vi "dfd_Lattice Coef Cluster Validation.vi"(8 "error in (no error)":errorcluster, 11 "Lattice coef":T2) -> (0 "error out":errorcluster, 1 "gain":dbl, 2 "v":dbl[](array[numeric]), 3 "k":dbl[](array[numeric]), 5 "lattice type":T1)   [LabVIEW 2017, in "NI_DigFilterLicensed.lvlib"]
uses:
  <vilib>/addons/Digital Filter Design/NI_DigFilterLicensed.lvlib
  <vilib>/addons/Digital Filter Design/_Objects.llb/DFD Filter Structure Type Selector.ctl
  <vilib>/addons/Digital Filter Design/_Misc.llb/dfd_Error Handlers (Multiple).vi
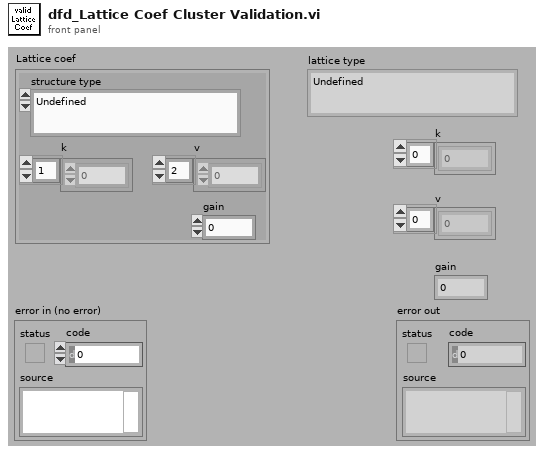
[diagram p1: front panel]
types:
  T1 = typedef "NI_DigFilterLicensed.lvlib/DFD Filter Structure Type Selector.ctl" = enum16{"Undefined", "FIR Direct Form", "FIR Direct Form Transposed", "FIR Symmetric", "FIR Antisymmetric", "IIR Direct Form I", "IIR Direct Form I Transposed", "IIR Direct Form II", "IIR Direct Form II Transposed", "IIR Cascaded Second Order Sections Form I", "IIR Cascaded Second Order Sections Form I Transposed", "IIR Cascaded Second Order Sections Form II", "IIR Cascaded Second Order Sections Form II Transposed", "Lattice Allpass (basic sections)", "Lattice Allpass (one multiplier sections)", "Lattice Allpass (normalized sections)", "Lattice AR (basic sections)", "Lattice AR (one multiplier sections)", "Lattice AR (normalized sections)", "Lattice MA (minimum phase)", "Lattice MA (maximum phase)", "Lattice ARMA (basic sections)", "Lattice ARMA (one multiplier sections)", "Lattice ARMA (normalized sections)"}
  T2 = cluster{"structure type":T1, "k":dbl[], "v":dbl[], "gain":dbl}
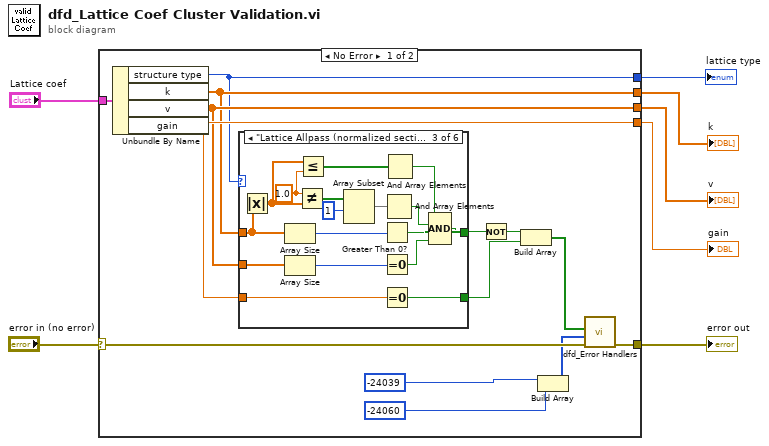
[diagram p0: block diagram]
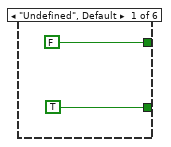
[diagram p2: hidden frame]
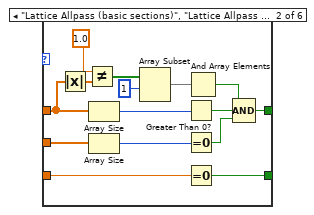
[diagram p3: hidden frame]
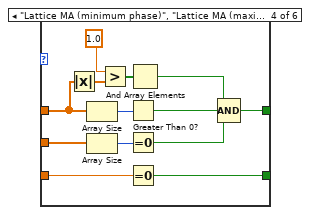
[diagram p4: hidden frame]
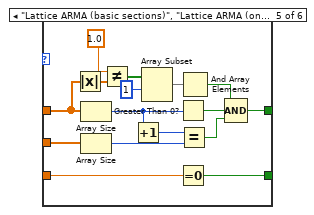
[diagram p5: hidden frame]
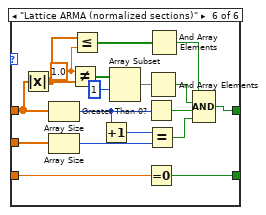
[diagram p6: hidden frame]
diagram:
  n1 = case shown="No Error" "error in (no error)" {
    selector: "error in (no error)" -> [w20 w103]
    tunnel: "Lattice coef" -> [w21 _]
    tunnel: [w19 w103] -> w5
    tunnel: [w18 _] -> w1
    tunnel: [w17 _] -> w2
    tunnel: [w16 _] -> w3
    tunnel: [w15 _] -> w4
    frame No Error {
      n2 = Unbundle By Name(w21) -> ("structure type"=w15:T1, "k"=w16:dbl[], "v"=w17:dbl[], "gain"=w18:dbl)
      n3 = case shown="\"Lattice Allpass (normalized sections)\", \"Lattice AR (normalized sections)\"" w15 {
        tunnel: w16 -> [_ w35 w52 w65 w82 w100]
        tunnel: w17 -> [_ w38 w55 w68 w84 w102]
        tunnel: w18 -> [_ w36 w53 w66 w83 w101]
        tunnel: [FALSE w28 w47 w57 w73 w93] -> w14
        tunnel: [TRUE w24 w43 w56 w69 w89] -> w11
        frame "Undefined", Default {
        }
        frame "Lattice Allpass (basic sections)", "Lattice Allpass (one multiplier sections)", "Lattice AR (basic sections)", "Lattice AR (one multiplier sections)" {
          n4 = Absolute Value(x=w35) -> (abs(x)=w33:dbl[])
          n5 = Not Equal?(x=1.0, y=w33) -> (x != y?=w27:bool[])
          n6 = Array Size(array=w35) -> (size(s)=w34:i32)
          n7 = Array Size(array=w38) -> (size(s)=w37:i32)
          n8 = Array Subset(array=w27, index=1) -> (w25:bool[])  [unwired: 1 in]
          n9 = Greater Than 0?(x=w34) -> (x > 0?=w30:bool)
          n10 = Equal To 0?(x=w37) -> (x = 0?=w31:bool)
          n11 = Equal To 0?(x=w36) -> (x = 0?=w24:bool)
          n12 = And Array Elements(Boolean array=w25) -> (logical AND=w29:bool)
          n13 = Compound Arithmetic op=AND(w29, w30, w31) -> (w28:bool)
        }
        frame "Lattice Allpass (normalized sections)", "Lattice AR (normalized sections)" {
          w41 = 1.0
          n14 = Absolute Value(x=w52) -> (abs(x)=w42:dbl[])
          n15 = Array Size(array=w52) -> (size(s)=w51:i32)
          n16 = Array Size(array=w55) -> (size(s)=w54:i32)
          n17 = Not Equal?(x=w41, y=w42) -> (x != y?=w46:bool[])
          n18 = Less Or Equal?(x=w42, y=w41) -> (x <= y?=w40:bool[])
          n19 = Array Subset(array=w46, index=1) -> (w44:bool[])  [unwired: 1 in]
          n20 = Greater Than 0?(x=w51) -> (x > 0?=w49:bool)
          n21 = Equal To 0?(x=w54) -> (x = 0?=w50:bool)
          n22 = Equal To 0?(x=w53) -> (x = 0?=w43:bool)
          n23 = And Array Elements(Boolean array=w44) -> (logical AND=w48:bool)
          n24 = And Array Elements(Boolean array=w40) -> (logical AND=w39:bool)
          n25 = Compound Arithmetic op=AND(w39, w48, w49, w50) -> (w47:bool)
        }
        frame "Lattice MA (minimum phase)", "Lattice MA (maximum phase)" {
          n26 = Absolute Value(x=w65) -> (abs(x)=w63:dbl[])
          n27 = Array Size(array=w65) -> (size(s)=w64:i32)
          n28 = Array Size(array=w68) -> (size(s)=w67:i32)
          n29 = Greater?(x=1.0, y=w63) -> (0:w61:bool[])
          n30 = Greater Than 0?(x=w64) -> (x > 0?=w59:bool)
          n31 = Equal To 0?(x=w67) -> (x = 0?=w60:bool)
          n32 = Equal To 0?(x=w66) -> (x = 0?=w56:bool)
          n33 = And Array Elements(Boolean array=w61) -> (logical AND=w58:bool)
          n34 = Compound Arithmetic op=AND(w58, w59, w60) -> (w57:bool)
        }
        frame "Lattice ARMA (basic sections)", "Lattice ARMA (one multiplier sections)" {
          n35 = Absolute Value(x=w82) -> (abs(x)=w81:dbl[])
          n36 = Array Size(array=w82) -> (size(s)=w76:i32)
          n37 = Array Size(array=w84) -> (size(s)=w77:i32)
          n38 = Not Equal?(x=1.0, y=w81) -> (x != y?=w72:bool[])
          n39 = Increment(x=w76) -> (x+1=w75:i32)
          n40 = Array Subset(array=w72, index=1) -> (w70:bool[])  [unwired: 1 in]
          n41 = Greater Than 0?(x=w76) -> (x > 0?=w78:bool)
          n42 = Equal To 0?(x=w83) -> (x = 0?=w69:bool)
          n43 = Equal?(x=w75, y=w77) -> (x = y?=w74:bool)
          n44 = And Array Elements(Boolean array=w70) -> (logical AND=w79:bool)
          n45 = Compound Arithmetic op=AND(w79, w78, w74) -> (w73:bool)
        }
        frame "Lattice ARMA (normalized sections)" {
          w87 = 1.0
          n46 = Absolute Value(x=w100) -> (abs(x)=w88:dbl[])
          n47 = Array Size(array=w100) -> (size(s)=w96:i32)
          n48 = Array Size(array=w102) -> (size(s)=w97:i32)
          n49 = Not Equal?(x=w87, y=w88) -> (x != y?=w92:bool[])
          n50 = Less Or Equal?(x=w88, y=w87) -> (x <= y?=w86:bool[])
          n51 = Increment(x=w96) -> (x+1=w95:i32)
          n52 = Array Subset(array=w92, index=1) -> (w90:bool[])  [unwired: 1 in]
          n53 = Greater Than 0?(x=w96) -> (x > 0?=w98:bool)
          n54 = Equal To 0?(x=w101) -> (x = 0?=w89:bool)
          n55 = Equal?(x=w95, y=w97) -> (x = y?=w94:bool)
          n56 = And Array Elements(Boolean array=w90) -> (logical AND=w99:bool)
          n57 = And Array Elements(Boolean array=w86) -> (logical AND=w85:bool)
          n58 = Compound Arithmetic op=AND(w85, w99, w98, w94) -> (w93:bool)
        }
      }
      n59 = Not(x=w14) -> (.not. x?=w13:bool)
      n60 = Build Array(w13, w11) -> (w12:bool[])
      n61 = Build Array(-24039 ("ERR_INVALID_LAT_COEF"), -24060 ("ERR_GAIN_NOT_ZERO")) -> (w10:i32[])
      n62 = call-poly <vilib>:"dfd_Error Handlers.vi"("error in (no error)"=w20, "error sources"=w10, "condition failed?"=w12) -> ("error out"=w19:errorcluster)  [unwired: 8 out]
    }
    frame Error {
    }
  }
  "error out" <- w5
  "lattice type" <- w4
  "k" <- w3
  "v" <- w2
  "gain" <- w1
